vi "test.vi"(7 "LabVIEW Web Service Request":refnum<class "Web Request.lvclass">) -> ()   [LabVIEW 2014]
uses:
  <vilib>/wsapi/Web Request.lvclass
  i3-sse-server.lvlib
  <vilib>/wsapi/Web Service.lvclass
panel:
  out "Error Out":errorcluster
  # "Use the Web Service Request input terminal to call the VIs on the Web Services palette. Do not remove it from the connector pane unless you don't need access to the palette."
  # "Each additional control wired to the connector pane will be available as an input in the URL. To include an indicator in terminal-mode output (the default setting), it must also be wired to the connector pane."
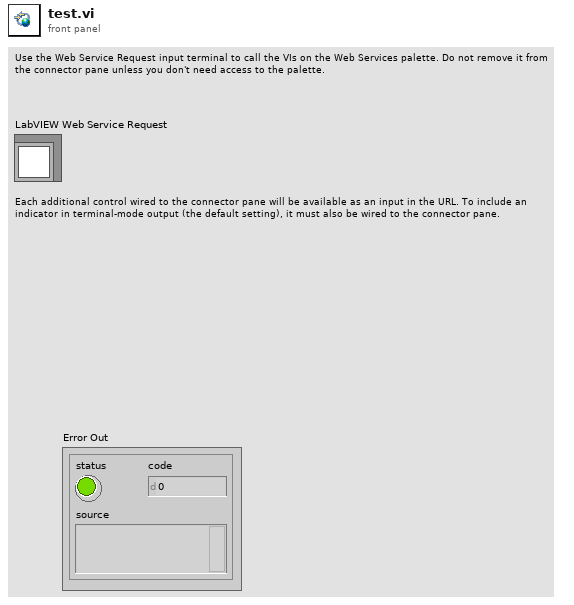
[diagram p1: front panel]
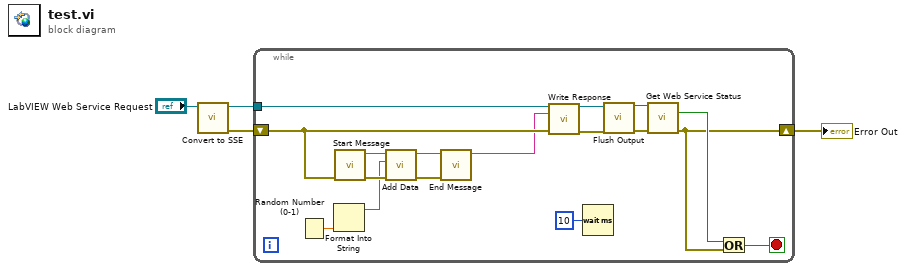
[diagram p0: block diagram]
diagram:
  n1 = call "Convert to SSE.vi"("LabVIEW Web Service Request In"="LabVIEW Web Service Request") -> ("Error Out"=w2:errorcluster, "LabVIEW Web Service Request Out"=w3:refnum<class "Web Request.lvclass">)  [unwired: 7 in, 2 out]
  n2 = while {
    tunnel: w3 -> [w20]
    shift-right: [w7] -> w1
    shift-left: w2 -> [w14]
    stop <- w6 stop-if-true
    n3 = Random Number (0-1)() -> (number: 0 to 1=w21:dbl)
    n4 = Format Into String(w21) -> (resulting string=w15:string)  [unwired: 3 in, 1 out]
    n5 = call "Start Message.vi"("Error In"=w14) -> ("Error Out"=w16:errorcluster, "Message Out"=w17:string)  [unwired: 9 in]
    n6 = call "Add Data.vi"("Error In"=w16, "Data"=w15, "Message In"=w17) -> ("Error Out"=w13:errorcluster, "Message Out"=w12:string)  [unwired: 7 in]
    n7 = call "End Message.vi"("Error In"=w13, "Message In"=w12) -> ("Message Out"=w11:string)  [unwired: 8 in, 1 out]
    n8 = call <vilib>:"Write Response.vi"("LabVIEW Web Service Request"=w20, "response string"=w11, "error in (no error)"=w14) -> ("LabVIEW Web Service Request out"=w19:refnum<class "Web Request.lvclass">, "error out"=w18:errorcluster)  [unwired: 11 in]
    n9 = Wait (ms)(milliseconds to wait=u32 10) -> ()  [unwired: 1 out]
    n10 = call <vilib>:"Flush Output.vi"("LabVIEW Web Service Request"=w19, "error in (no error)"=w18) -> ("LabVIEW Web Service Request out"=w9:refnum<class "Web Request.lvclass">, "error out"=w10:errorcluster)  [unwired: 12 in]
    n11 = call <vilib>:"Get Web Service Status.vi"("LabVIEW Web Service"=w9, "error in (no error)"=w10) -> ("service stopping?"=w8:bool, "error out"=w7:errorcluster)  [unwired: 11 in, 1 out]
    n12 = Or(x=w8, y=w7) -> (x .or. y?=w6:bool)
  }
  "Error Out" <- w1
